vi "Add Extra position_tester.vi"() -> ()   [LabVIEW 2022 SP3]
panel:
  in  "Near Constant":dbl[][](array[numeric])=[[-500.0, 7.0], [-400.0, 7.2], [-300.0, 8.0], [-200.0, 7.5], [-100.0, 7.2], [0.0, 8.0], [100.0, 7.5], [200.0, 7.0], [300.0, 8.0], [400.0, 7.2], [500.0, 7.3]]
  in  "Double gaussian":dbl[][](array[numeric])=[[-500.0, 0.0], [-400.0, 50.0], [-300.0, 100.0], [-200.0, 80.0], [-100.0, 20.0], [0.0, 0.0], [100.0, 60.0], [200.0, 150.0], [300.0, 300.0], [400.0, 100.0], [500.0, 50.0]]
  out "Numeric":i32=16
  in  "single unsemetrical peak":dbl[][](array[numeric])=[[-500.0, 0.0], [-400.0, 2.0], [-300.0, 5.0], [-200.0, 20.0], [-100.0, 50.0], [0.0, 100.0], [100.0, 500.0], [200.0, 10.0], [300.0, 0.0], [400.0, 0.0], [500.0, 0.0]]
  out "appended array":dbl[][](array[numeric])=[[-500.0, 0.0], [-400.0, 2.0], [-300.0, 5.0], [-200.0, 20.0], [-100.0, 50.0], [0.0, 100.0], [12.5, 150.0], [25.0, 200.0], [37.5, 250.0], [50.0, 300.0], [62.5, 350.0], [75.0, 400.0], [87.5, 450.0], [100.0, 500.0], [106.25, 469.375], [112.5, 438.75], [118.75, 408.125], [125.0, 377.5], [137.5, 316.25], [150.0, 255.0], [162.5, 193.75], [175.0, 132.5], [187.5, 71.25], [200.0, 10.0], [300.0, 0.0], [400.0, 0.0], [500.0, 0.0], [-50.0, 75.0]]
  in  "stop":bool
  in  "Another point":bool
  out "XY Graph":T1(graph)={"Positions   Concentration"=[-500.0, -400.0, -300.0, -200.0, -100.0, 0.0, 12.5, 25.0, 37.5, 50.0, 62.5, 75.0, 87.5, 100.0, 106.25, 112.5, 118.75, 125.0, 137.5, 150.0, 162.5, 175.0, 187.5, 200.0, 300.0, 400.0, 500.0], "Positions   Concentration"=[0.0, 2.0, 5.0, 20.0, 50.0, 100.0, 150.0, 200.0, 250.0, 300.0, 350.0, 400.0, 450.0, 500.0, 469.375, 438.75, 408.125, 377.5, 316.25, 255.0, 193.75, 132.5, 71.25, 10.0, 0.0, 0.0, 0.0]}
  in  "single gaussian":dbl[][](array[numeric])=[[-500.0, 0.0], [-400.0, 0.0], [-300.0, 30.0], [-200.0, 80.0], [-100.0, 200.0], [0.0, 150.0], [100.0, 50.0], [200.0, 10.0], [300.0, 0.0], [400.0, 0.0], [500.0, 0.0]]
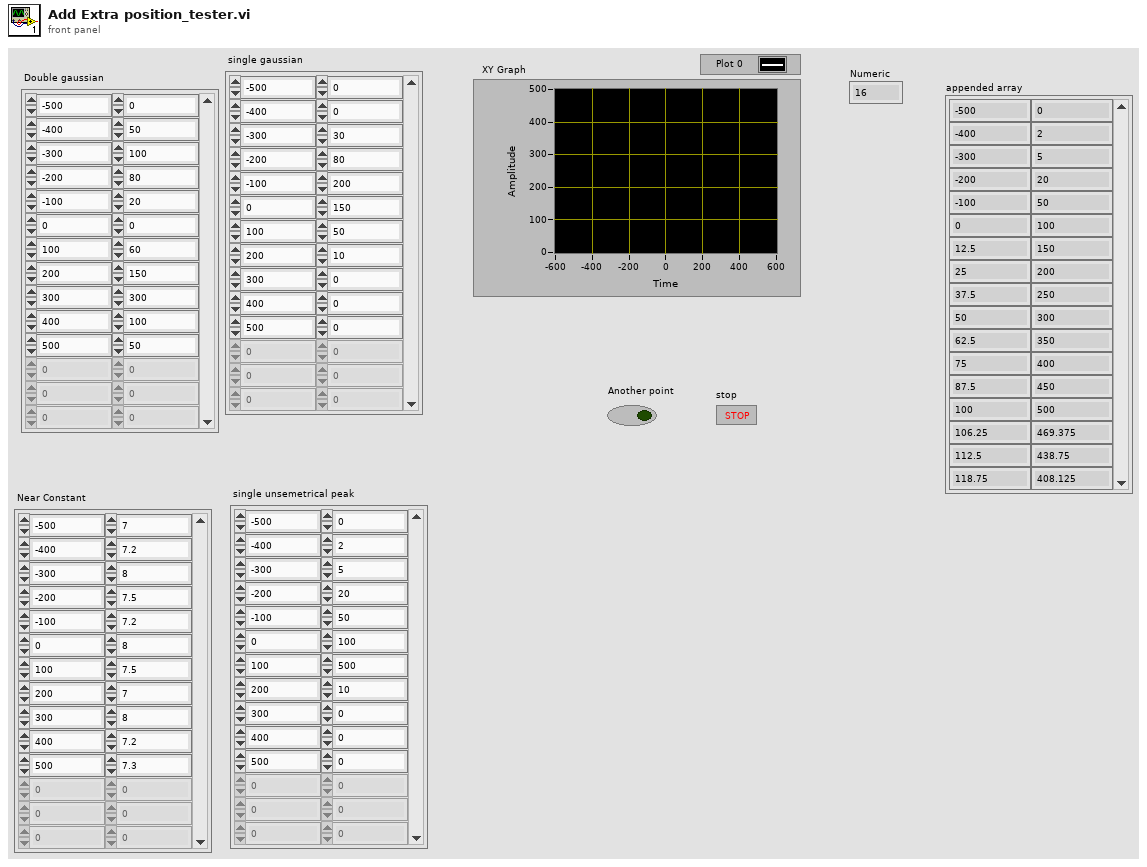
[diagram p1: front panel]
types:
  T1 = cluster{"Positions   Concentration":dbl[], "Positions   Concentration":dbl[]}
  T2 = cluster{"sorted array":dbl[], "sorted array":dbl[]}
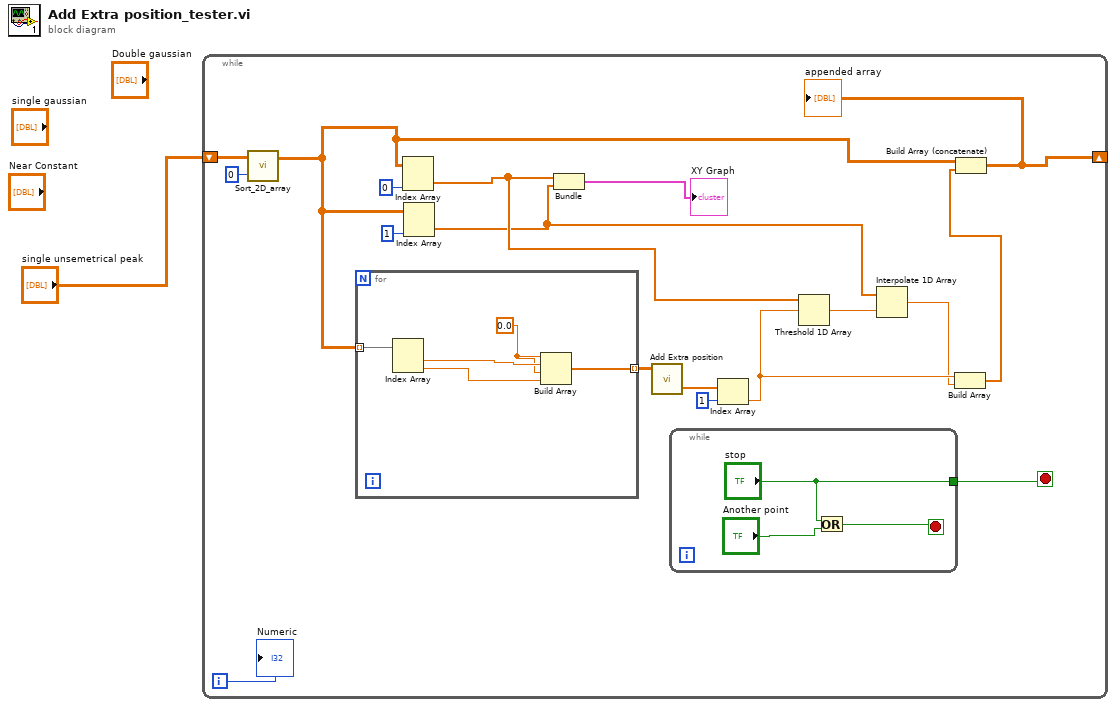
[diagram p0: block diagram]
diagram:
  n1 = while {
    shift-right: [w4] -> _
    shift-left: "single unsemetrical peak" -> [w13]
    i -> [w3]
    stop <- w2 stop-if-true
    n2 = call "Sort_2D_array.vi"("Column index to sort on"=0, "unsorted array"=w13) -> ("sorted array"=w11:dbl[][])  [unwired: 1 out]
    n3 = for {
      tunnel: w11 -> [w27] mode=indexing
      tunnel: [w23] -> w19 mode=indexing
      w25 = 0.0 ("element")
      n4 = Index Array(array=w27) -> (element #1=w26:dbl, element #2=w24:dbl)  [unwired: 2 in]
      n5 = Build Array(w25, w26, w25, w24) -> (w23:dbl[])
    }
    n6 = Index Array(array=w11, index (col)=0 ("disabled index (col)")) -> (element=w10:dbl[])  [unwired: 1 in]
    n7 = Index Array(array=w11, index (col)=1 ("disabled index (col)")) -> (element=w8:dbl[])  [unwired: 1 in]
    n8 = Bundle("sorted array"=w10, "sorted array"=w8) -> (→"XY Graph":T2)  [unwired: 1 in]
    n9 = call "Add Extra position.vi"("Positions"=w19) -> ("Additional Point"=w15:dbl[])  [unwired: 3 in]
    n10 = while {
      tunnel: ["stop"] -> w2
      stop <- w21 stop-if-true
      n11 = Or(x="stop", y="Another point") -> (x .or. y?=w21:bool)
    }
    n12 = Index Array(array=w15, index=1) -> (element=w7:dbl)
    n13 = Threshold 1D Array(2:w7, 3:w10) -> (0:w9:dbl)  [unwired: 1 in]
    n14 = Interpolate 1D Array(1:w9, 2:w8) -> (0:w6:dbl)
    n15 = Build Array(w7, w6) -> (w5:dbl[])
    n16 = Build Array (concatenate)(w11, w5) -> (w4:dbl[][])
    "appended array" <- w4
    "Numeric" <- w3
  }
